vi "Receive Wfm.vi"(6 "Receive Time":timestamp, 8 "error in (no error)":errorcluster, 9 "Wfm Properties":T1, 10 "Data in":dbl[](array[numeric]), 11 "Waveform Receive in":refnum<class "Waveform Receive.lvclass">) -> (0 "error out":errorcluster, 2 "Data out":dbl[](array[numeric]), 3 "Waveform Receive out":refnum<class "Waveform Receive.lvclass">)   [LabVIEW 2015, in "Waveform Receive.lvclass"]
uses:
  Waveform Receive.lvclass
  <vilib>/NI Veristand/Custom Device Waveform API/Waveform properties.ctl
  <vilib>/NI Veristand/Custom Device API/Waveform Data Reference.ctl
  Waveform Receive.lvclass/Waveform Receive.ctl
  <vilib>/NI Veristand/Custom Device API/Custom Device API.lvlib
  <vilib>/NI Veristand/Custom Device Waveform API/NI_VS Custom Device Waveform API.lvlib
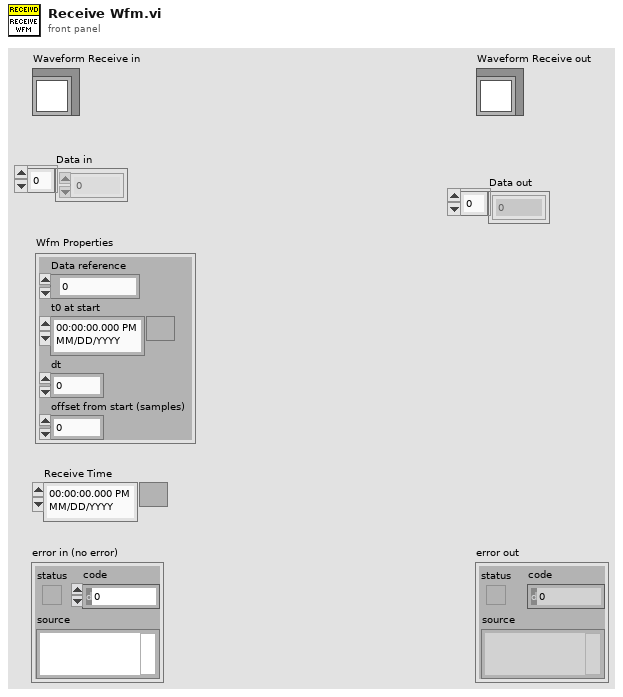
[diagram p1: front panel]
types:
  T1 = typedef "NI_VS Custom Device Waveform API.lvlib/Waveform properties.ctl" = cluster{"Data reference":T2, "t0 at start":timestamp, "dt":dbl, "offset from start (samples)":u64}
  T2 = typedef "Custom Device API.lvlib/Waveform Data Reference.ctl" = i32
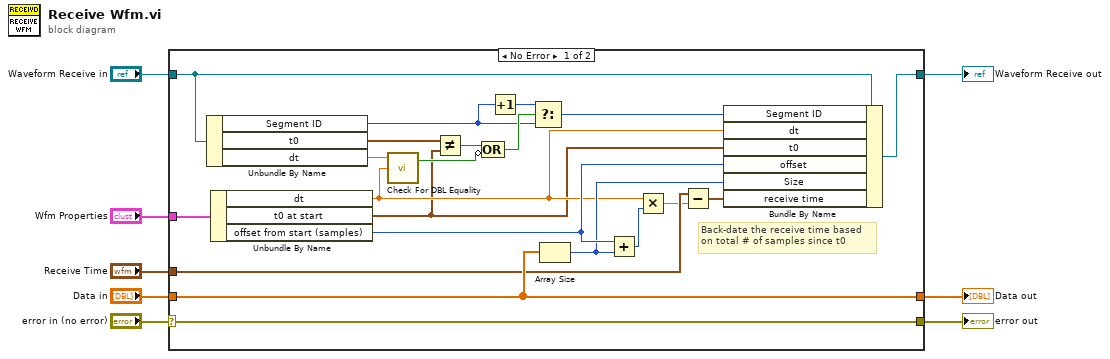
[diagram p0: block diagram]
diagram:
  n1 = case shown="No Error" "error in (no error)" {
    selector: "error in (no error)" -> [w29 w32]
    tunnel: [w29 w32] -> w7
    tunnel: [w28 w31] -> w5
    tunnel: "Waveform Receive in" -> [w27 w31]
    tunnel: "Receive Time" -> [w15 _]
    tunnel: "Wfm Properties" -> [w26 _]
    tunnel: "Data in" -> [w19 w30]
    tunnel: [w19 w30] -> w1
    frame No Error {
      # "Back-date the receive time based\non total # of samples since t0"
      n2 = Unbundle By Name(w27) -> ("Segment ID"=w21:u64, "t0"=w25:timestamp, "dt"=w12:dbl)
      n3 = Unbundle By Name(w26) -> ("dt"=w11:dbl, "t0 at start"=w9:timestamp, "offset from start (samples)"=w18:u64)
      n4 = call "Check For DBL Equality.vi"("n2"=w11, "n1"=w12) -> ("equal?"=w10:bool)  [unwired: 2 in]
      n5 = Not Equal?(x=w25, y=w9) -> (x != y?=w24:bool)
      n6 = Compound Arithmetic op=OR(w24, invert w10) -> (w23:bool)
      n7 = Increment(x=w21) -> (x+1=w22:u64)
      n8 = Select(t=w22, s=w23, f=w21) -> (s? t:f=w20:u64)
      n9 = Array Size(array=w19) -> (size(s)=w17:i32)
      n10 = Add(x=w18, y=w17) -> (x+y=w16:u64)
      n11 = Multiply(x=w11, y=w16) -> (x*y=w14:dbl)
      n12 = Subtract(x=w15, y=w14) -> (x-y=w13:timestamp)
      n13 = Bundle By Name(cluster=w27, "Segment ID"=w20, "dt"=w11, "t0"=w9, "offset"=w18, "Size"=w17, "receive time"=w13) -> (w28:refnum<class "Waveform Receive.lvclass">)
    }
    frame Error {
    }
  }
  "error out" <- w7
  "Waveform Receive out" <- w5
  "Data out" <- w1
